vi "UnpackedFlatVectorToMatrix.vi"(9 "FlatValues":dbl[](array[numeric]), 10 "colDim":u32, 11 "rowDim":u32) -> (3 "Matrix":dbl[][](array[numeric]))   [LabVIEW 2020]
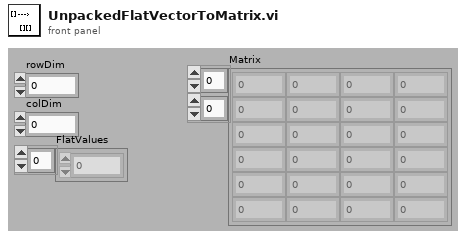
[diagram p1: front panel]
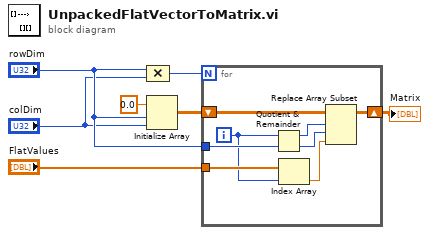
[diagram p0: block diagram]
diagram:
  n1 = Compound Arithmetic op=MULTIPLY("rowDim", "colDim") -> (w7:u32)
  n2 = Initialize Array(0.0 ("element"), "rowDim", "colDim") -> (w6:dbl[][])
  n3 = for {
    N: w7 -> [_]
    shift-right: [w14] -> w4
    shift-left: w6 -> [w15]
    tunnel: "rowDim" -> [w13]
    tunnel: "FlatValues" -> [w10]
    i -> [w8]
    n4 = Quotient & Remainder(x=w8, y=w13) -> (x-y*floor(x/y)=w12:u32, floor(x/y)=w11:u32)
    n5 = Index Array(array=w10, index=w8) -> (element=w9:dbl)
    n6 = Replace Array Subset(array=w15, new element=w9, index (row)=w12, index (col)=w11) -> (w14:dbl[][])
  }
  "Matrix" <- w4
